vi "write input registers.vi"(7 "Regs to Write":bool[](array[boolean]), 8 "error in (no error)":errorcluster, 9 "Channel Data":T1[](array[typedef]), 10 "Values":dbl[](array[numeric]), 11 "Modbus slave in":refnum<class "Modbus Slave.lvclass">) -> (0 "error out":errorcluster)   [LabVIEW 2015, in "Modbus Master Engine.lvlib"]
uses:
  Modbus Master Engine.lvlib
  Shared/Controls/Data Model/Channel.ctl
  System Explorer/SubVIs/Modbus Type.ctl
  <vilib>/NI Veristand/Custom Device API/Custom Device Channel Type.ctl
  Shared/Controls/Data Model/Mapping.ctl
  Shared/Controls/Data Model/DataType.ctl
  <vilib>/NI Veristand/Custom Device API/Custom Device Item Ref.ctl
  Modbus API.lvlibp/API/Slave/Modbus Slave.lvclass
  Shared/Modbus Master Shared.lvlib
  <vilib>/NI VeriStand/Custom Device API/Custom Device API.lvlib
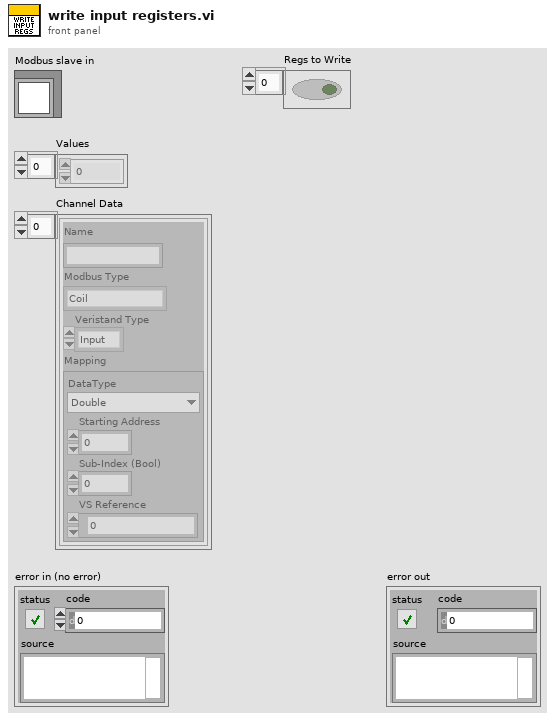
[diagram p1: front panel]
types:
  T1 = typedef "Modbus Master Shared.lvlib/Channel.ctl" = cluster{"Name":string, "Modbus Type":T2, "Veristand Type":T3, "Mapping":T4}
  T2 = typedef "Modbus Master Shared.lvlib/Modbus Type.ctl" = enum16{"Coil", "Discrete Input", "Holding Register", "Input Register"}
  T3 = typedef "Custom Device API.lvlib/Custom Device Channel Type.ctl" = enum16{"Input", "Output"}
  T4 = typedef "Modbus Master Shared.lvlib/Mapping.ctl" = cluster{"DataType":T5, "Starting Address":u16, "Sub-Index (Bool)":u16, "VS Reference":T6}
  T5 = typedef "Modbus Master Shared.lvlib/DataType.ctl" = enum16{"Double", "Single", "I64", "I32", "I16", "I8", "U64", "U32", "U16", "U8", "Boolean"}
  T6 = typedef "Custom Device API.lvlib/Custom Device Item Ref.ctl" = u64
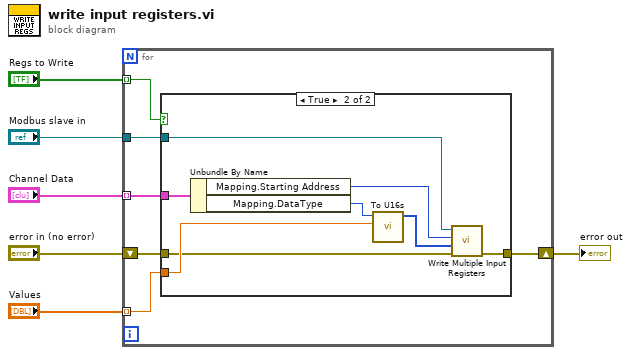
[diagram p0: block diagram]
diagram:
  n1 = for {
    tunnel: "Modbus slave in" -> [w12]
    tunnel: "Values" -> [w9] mode=indexing
    shift-right: [w10] -> w3
    shift-left: "error in (no error)" -> [w11]
    tunnel: "Regs to Write" -> [w8] mode=indexing
    tunnel: "Channel Data" -> [w7] mode=indexing
    n2 = case shown="True" w8 {
      tunnel: w12 -> [_ w18]
      tunnel: w11 -> [w13 w15]
      tunnel: [w13 w14] -> w10
      tunnel: w9 -> [_ w19]
      tunnel: w7 -> [_ w21]
      frame False {
      }
      frame True {
        n3 = Unbundle By Name(w21) -> ("Mapping.Starting Address"=w17:u16, "Mapping.DataType"=w20:T5)
        n4 = call "To U16s.vi"("Numeric"=w19, "DataType"=w20) -> ("Array"=w16:u16[])  [unwired: 9 in]
        n5 = call-dynamic "Write Multiple Input Registers.vi"("error in"=w15, "input registers to write"=w16, "starting address"=w17, "Modbus slave in"=w18) -> ("error out"=w14:errorcluster)  [unwired: 6 in, 1 out]
      }
    }
  }
  "error out" <- w3
